vi "Create_Trajectory_All_WP_Meters_To_Units.vi"(10 "Units Selector":T2, 11 "WayPoints_M":T1[](array[typedef]) {"WEIGHT" format="%13.3f"; "ANGLE" format="%13.3f"; "Y" format="%13.3f"; "X" format="%13.3f"}) -> (3 "outWayPoints_UNITS":T1[](array[typedef]) {"WEIGHT" format="%13.3f"; "ANGLE" format="%13.3f"; "Y" format="%13.3f"; "X" format="%13.3f"})   [LabVIEW 2019]
uses:
  <vilib>/Rock Robotics/WPI/ThirdParty/JAS_Junk/TrajLib/DISPLAY_WEIGHTED_WAYPOINT.ctl
  TrajCreateUnitsENUM.ctl
  <vilib>/Rock Robotics/WPI/ThirdParty/JAS_Junk/TrajLib/Conv_Meters_Inches.vi
  <vilib>/Rock Robotics/WPI/ThirdParty/JAS_Junk/TrajLib/Conv_Meters_Feet.vi
  <vilib>/Rock Robotics/WPI/ThirdParty/JAS_Junk/TrajLib/Trajectory_Library.lvlib
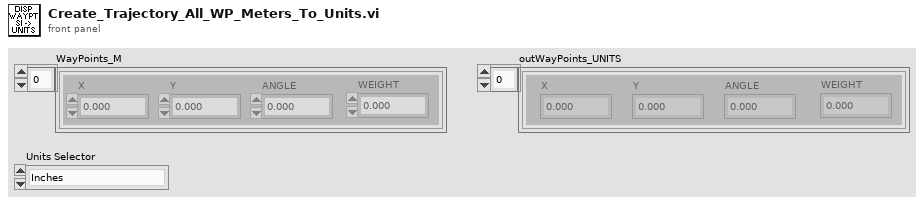
[diagram p1: front panel]
types:
  T1 = typedef "Trajectory_Library.lvlib/DISPLAY_WEIGHTED_WAYPOINT.ctl" = cluster{"X":dbl, "Y":dbl, "ANGLE":dbl, "WEIGHT":dbl}
  T2 = typedef "TrajCreateUnitsENUM.ctl" = enum16{"Inches", "Feet", "Centimeters", "Meters"}
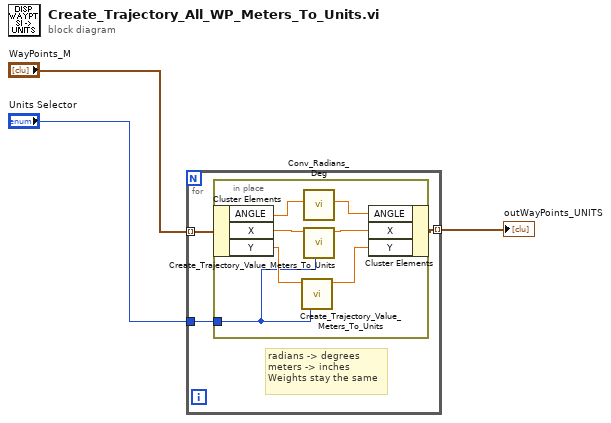
[diagram p0: block diagram]
diagram:
  n1 = for {
    tunnel: "WayPoints_M" -> [w6] mode=indexing
    tunnel: [w5] -> w1 mode=indexing
    tunnel: "Units Selector" -> [w4]
    # "radians -> degrees\nmeters -> inches\nWeights stay the same"
    n2 = in-place {
      in-place-border: w4 -> [w7]
      n3 = in-place-cluster #1(w6) -> ("ANGLE"=w8:dbl, "X"=w13:dbl, "Y"=w11:dbl)
      n4 = call "Create_Trajectory_Value_Meters_To_Units.vi"("Units Selector"=w7, "Meters"=w11) -> ("Units"=w10:dbl)  [unwired: 9 in]
      n5 = call <vilib>:"Conv_Radians_Deg.vi"("Radians"=w8) -> ("Degrees"=w9:dbl)  [unwired: 10 in]
      n6 = call "Create_Trajectory_Value_Meters_To_Units.vi"("Units Selector"=w7, "Meters"=w13) -> ("Units"=w12:dbl)  [unwired: 9 in]
      n7 = in-place-cluster #1("ANGLE"=w9, "X"=w12, "Y"=w10) -> (w5:T1)
    }
  }
  "outWayPoints_UNITS" <- w1
